vi "全局.vi"() -> ()   [LabVIEW 2015]
panel:
  out "停止":bool
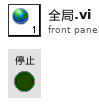
[diagram p1: front panel]
diagram:
